vi "data.vi"(7 "LVWSR":refnum<class "Web Request.lvclass">) -> ()   [LabVIEW 2016]
uses:
  <vilib>/wsapi/Web Request.lvclass
  <vilib>/MSR Consulting, LLC/General Reuse/Data/Data.lvclass
  Controller/gController.lvclass
panel:
  out "data":string="{}"
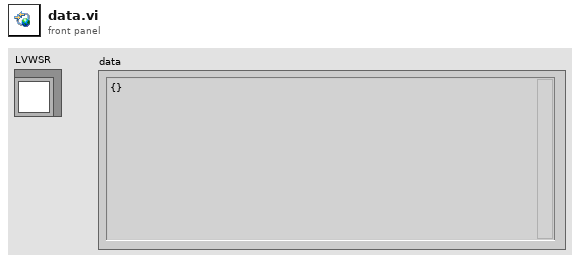
[diagram p1: front panel]
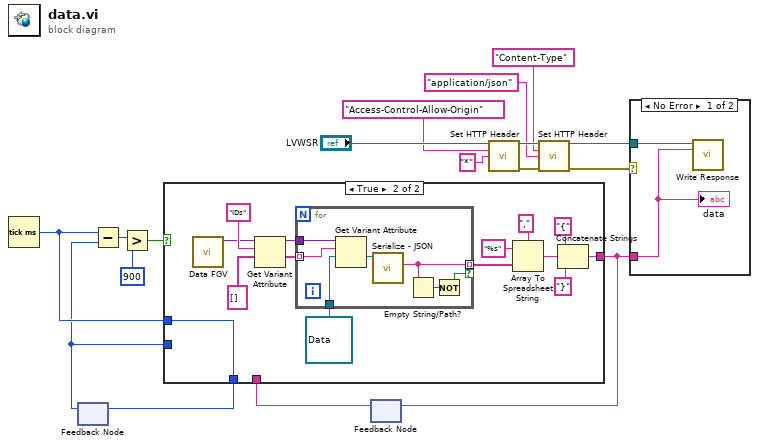
[diagram p0: block diagram]
diagram:
  n1 = Tick Count (ms)() -> (millisecond timer value=w3:u32)
  n2 = feedback #1() -> (w1:u32)  [unwired: 1 in]
  n3 = Subtract(x=w3, y=w1) -> (x-y=w8:u32)
  n4 = Greater?(x=w8, y=u32 900) -> (0:w4:bool)
  n5 = feedback #2() -> (w5:string)  [unwired: 1 in]
  n6 = case shown="True" w4 {
    tunnel: [w19 w22] -> w6
    tunnel: w5 -> [w19 _]
    tunnel: w3 -> [_ w20]
    tunnel: [w18 w20] -> w2
    tunnel: w1 -> [w18 _]
    frame False {
    }
    frame True {
      n7 = call "Data FGV.vi"() -> ("Data"=w21:variant)  [unwired: 10 in, 1 out]
      n8 = Get Variant Attribute(Variant=w21, name="IDs", default value (empty Variant)=string[] []) -> (duplicate Variant=w30:variant, value=w31:string[])  [unwired: 1 in, 2 out]
      n9 = for {
        tunnel: w31 -> [w40] mode=indexing
        tunnel: w30 -> [w39]
        tunnel: refnum<class "Data.lvclass"> refnum ("Base Data Lib:Data") -> [w38]
        tunnel: [w36] -> w23 mode=indexing if=w34
        n10 = Get Variant Attribute(Variant=w39, name=w40, default value (empty Variant)=w38) -> (value=w37:refnum<class "Data.lvclass">)  [unwired: 1 in, 3 out]
        n11 = call-dynamic "Serialize - JSON.vi"("Data in"=w37) -> ("Serialized JSON"=w36:string)  [unwired: 8 in, 2 out]
        n12 = Empty String/Path?(string/path=w36) -> (empty?=w35:bool)
        n13 = Not(x=w35) -> (.not. x?=w34:bool)
      }
      n14 = Array To Spreadsheet String(delimiter (Tab)=",", array=w23, 3:"%s" ("format string")) -> (spreadsheet string=w26:string)
      n15 = Concatenate Strings("{" ("string"), w26, "}" ("string")) -> (w22:string)
    }
  }
  n16 = feedback-in #1(w2) -> ()
  n17 = feedback-in #2(w6) -> ()
  n18 = call <vilib>:"Set HTTP Header.vi"("LabVIEW Web Service Request"="LVWSR", "header"="Access-Control-Allow-Origin", "header value"="*") -> ("LabVIEW Web Service Request out"=w16:refnum<class "Web Request.lvclass">, "error out"=w15:errorcluster)  [unwired: 11 in]
  n19 = call <vilib>:"Set HTTP Header.vi"("LabVIEW Web Service Request"=w16, "header"="Content-Type", "header value"="application/json", "error in (no error)"=w15) -> ("LabVIEW Web Service Request out"=w9:refnum<class "Web Request.lvclass">, "error out"=w10:errorcluster)  [unwired: 10 in]
  n20 = case shown="No Error" w10 {
    tunnel: w9 -> [w42 _]
    tunnel: w6 -> [w41 _]
    frame No Error {
      n21 = call <vilib>:"Write Response.vi"("LabVIEW Web Service Request"=w42, "response string"=w41) -> ()  [unwired: 12 in, 2 out]
      "data" <- w41
    }
    frame Error {
    }
  }
